vi "DataAcqisitionFormFile(SubVI).vi"(11 "file path (dialog if empty)":path) -> (0 "error out":errorcluster, 6 "XY Graph":cluster{dbl[], dbl[]}[](graph))   [LabVIEW 2019]
uses:
  <vilib>/Utility/file.llb/Read Delimited Spreadsheet (DBL).vi
  Global.vi
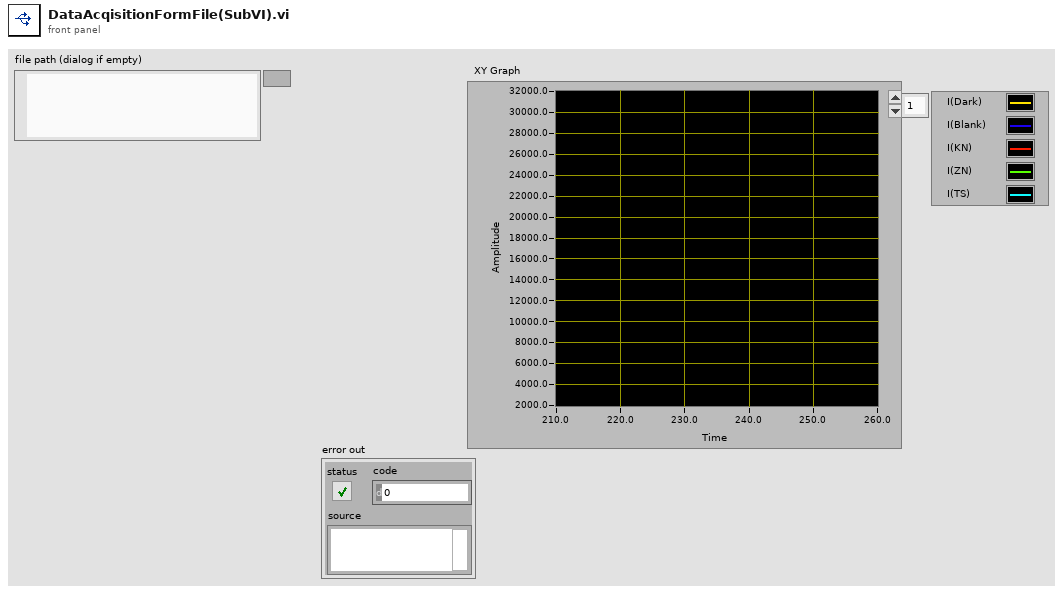
[diagram p1: front panel]
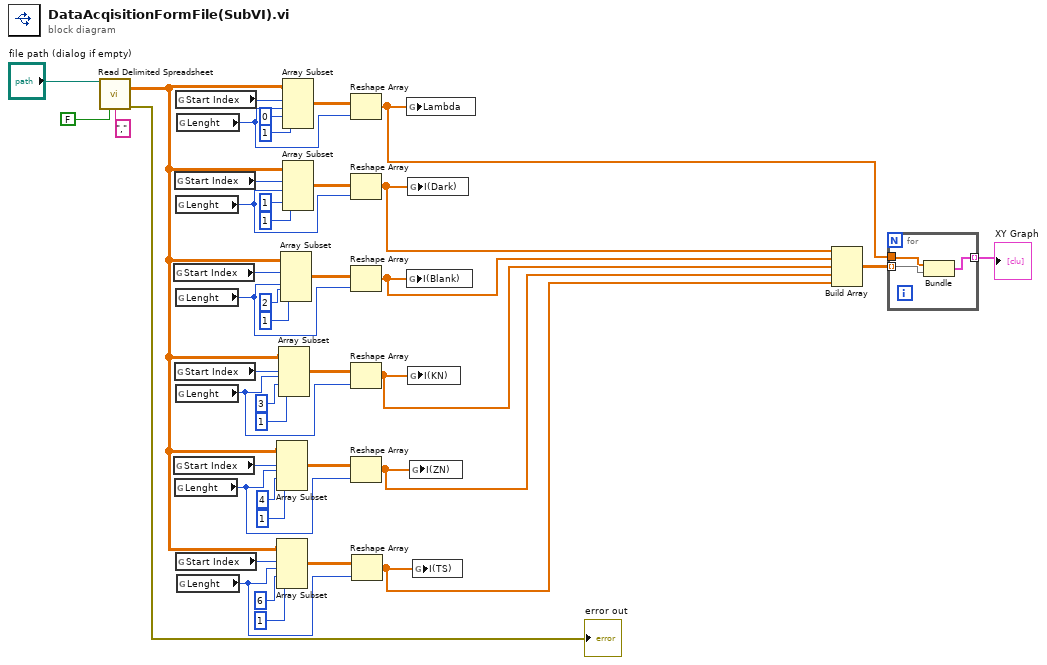
[diagram p0: block diagram]
diagram:
  n1 = call-poly <vilib>:"Read Delimited Spreadsheet.vi"("file path (dialog if empty)"="file path (dialog if empty)", "transpose? (F)"=FALSE, "delimiter (\\t)"="," ("delimiter (\\t)")) -> ("all rows"=w30:dbl[][], "error out"=→"error out":errorcluster)  [unwired: 7 in, 4 out]
  n2 = global read "Global.vi" "Start Index"() -> (w16:i32)
  n3 = global read "Global.vi" "Start Index"() -> (w14:i32)
  n4 = global read "Global.vi" "Start Index"() -> (w18:i32)
  n5 = global read "Global.vi" "Start Index"() -> (w15:i32)
  n6 = global read "Global.vi" "Lenght"() -> (w10:i32)
  n7 = global read "Global.vi" "Start Index"() -> (w20:i32)
  n8 = global read "Global.vi" "Lenght"() -> (w17:i32)
  n9 = global read "Global.vi" "Lenght"() -> (w9:i32)
  n10 = global read "Global.vi" "Lenght"() -> (w12:i32)
  n11 = global read "Global.vi" "Start Index"() -> (w13:i32)
  n12 = global read "Global.vi" "Lenght"() -> (w19:i32)
  n13 = global read "Global.vi" "Lenght"() -> (w11:i32)
  n14 = Array Subset(array=w30, index (row)=w14, length (row)=w10, index (col)=4 ("index"), length (col)=1 ("length")) -> (w21:dbl[][])
  n15 = Array Subset(array=w30, index (row)=w13, length (row)=w11, index (col)=6 ("index"), length (col)=1 ("length")) -> (w29:dbl[][])
  n16 = Array Subset(array=w30, index (row)=w15, length (row)=w12, index (col)=3 ("index"), length (col)=1 ("length")) -> (w22:dbl[][])
  n17 = Array Subset(array=w30, index (row)=w16, length (row)=w9, index (col)=2 ("index"), length (col)=1 ("length")) -> (w23:dbl[][])
  n18 = Array Subset(array=w30, index (row)=w20, length (row)=w19, index (col)=0 ("index"), length (col)=1 ("length")) -> (w25:dbl[][])
  n19 = Array Subset(array=w30, index (row)=w18, length (row)=w17, index (col)=1 ("index"), length (col)=1 ("length")) -> (w24:dbl[][])
  n20 = Reshape Array(w25, w19) -> (w6:dbl[])
  n21 = Reshape Array(w24, w17) -> (w5:dbl[])
  n22 = Reshape Array(w23, w9) -> (w4:dbl[])
  n23 = Reshape Array(w22, w12) -> (w3:dbl[])
  n24 = Reshape Array(w21, w10) -> (w2:dbl[])
  n25 = Reshape Array(w29, w11) -> (w1:dbl[])
  n26 = global write "Global.vi" "Lambda"(w6) -> ()
  n27 = global write "Global.vi" "I(Blank)"(w4) -> ()
  n28 = global write "Global.vi" "I(Dark)"(w5) -> ()
  n29 = global write "Global.vi" "I(KN)"(w3) -> ()
  n30 = global write "Global.vi" "I(ZN)"(w2) -> ()
  n31 = global write "Global.vi" "I(TS)"(w1) -> ()
  n32 = Build Array(w5, w4, w3, w2, w1) -> (w8:dbl[][])
  n33 = for {
    tunnel: w8 -> [w46] mode=indexing
    tunnel: [w45] -> w7 mode=indexing
    tunnel: w6 -> [w44]
    n34 = Bundle(w44, w46) -> (w45:cluster{dbl[], dbl[]})  [unwired: 1 in]
  }
  "XY Graph" <- w7
